vi "Main Editor UI.vi"() -> ()   [LabVIEW 2013, in "shared memory editor node.lvclass"]
doc: "This is the main view for configuration the behavior of a module in the DCAF standard editor."
uses:
  shared memory editor node.lvclass
  <vilib>/NI/Configuration Framework/Node/NodeRef.ctl
  <vilib>/NI/Configuration Framework/Node/NISE_CEF_Node.lvclass
  <vilib>/NI/AMC/Message Queue.ctl
  <vilib>/NI/AMC/Message.ctl
  <vilib>/NI/Tools/Keyed Array/KeyedArray.ctl
  <vilib>/NI/Configuration Framework/Node/UserEventRef.ctl
  <vilib>/NI/Configuration Framework/Controls/EventCluster.ctl
  <vilib>/NI/DCAF UI Toolkit/Controls/Configure.ctl
  <vilib>/NI/DCAF UI Toolkit/Controls/Add.ctl
  <vilib>/NI/DCAF UI Toolkit/Controls/Remove.ctl
  <vilib>/NI/Configuration Framework/Node/StopEvent.ctl
  <vilib>/NI/Configuration Framework/Node/RefreshUIEvent.ctl
  <vilib>/NI/Configuration Framework/Node/CacheState.ctl
  <vilib>/NI/Configuration Framework/Node/NodeChangeEvent.ctl
  <vilib>/NI/Tag Bus/tag/Data Type.ctl
  Permissions Enum.ctl
  <vilib>/NI/DCAF/Tag Editor Core/Table API/Available Tag Menu/channel action event.ctl
  <vilib>/NI/DCAF/Tag Editor Core/Table API/Available Tag Menu/dialog output action.ctl
  <vilib>/NI/Tag Bus Module Framework/channel/TBM channel.lvclass
  <vilib>/NI/Tag Bus/tag/tag descriptor.lvclass
  <vilib>/NI/DCAF/Tag Editor Core/Table API/Table Manager/Call Back Ref Type Def.ctl
  <vilib>/NI/DCAF/Tag Editor Core/Configuration Editor/Classes/Engine Parent/Engine Parent Editor Node.lvclass
  <vilib>/NI/DCAF/Tag Editor Core/Configuration Editor/Classes/Module editor node/module editor node.lvclass
  <vilib>/NI/DCAF/Tag Editor Core/Table API/Table Manager/references.ctl
  <vilib>/NI/DCAF/Tag Editor Core/Table API/Listbox/Multi Column Listbox.lvclass
  <vilib>/Utility/miscctls.llb/LVPositionTypeDef.ctl
  <vilib>/NI/DCAF/Tag Editor Core/Configuration Editor/Classes/Engine Parent/read engine configuration.vi
  <vilib>/NI/Configuration Framework/NISE_CEF_TreeControl.lvlib
  <vilib>/NI/Tools/Keyed Array/Tools_KeyedArray.lvlib
  <vilib>/NI/AMC/AMC.lvlib
  <vilib>/NI/DCAF/Tag Editor Core/Table API/Table Manager.lvlib
  <vilib>/NI/DCAF/Tag Editor Core/Table API/Table Manager/Table Manager.lvclass
  <vilib>/NI/DCAF UI Toolkit/Controls/DCAF UI Elements.lvlib
panel:
  in  "user event out":refnum<user-event>
  in  "Permissions":T1
  in  "data type":T2
  in  "node change":T3
  in  "cache state":T4
  in  "refresh UI":T5
  in  "stop event":T6
  in  "Tab Control":T7(tab)
  in  "Remove Button":T8
  in  "Add Button":T9
  in  "Table":i32(listbox)
  in  "settings":T10
  in  "output file string":string caption="output file string (data engine input)"
  in  "input file string":string caption="input file string (data engine output)"
  in  "name string":string caption="name string (optional)"
  in  "C header file directory":path
  in  "C header":bool
  in  "user event":T11
  in  "main queue":T12
  in  "node ref":T13
  # "Directories relative to engine root (/dev/shm/<EngineName>)"
  # "It is recommended that directory names be chosen to reflect the perspective of an the external process or application that accesses the file in shared memory.\n\nExample: A C application running in parallel to the DCAF based LabVIEW Real-Time EXE will view any folder that it writes to (which are read by the data engine) to be an \"output\" folder."
  # "C Header File Generation"
  # "Generate a C header file in a \"C header file directory\" which contains shared memory mapping information for use in C applications. The default C header file name will use the configuration file name and add optional user \"name string\" text: \n\nConfigurationFileName<_NameString>.h\n\nNote: The user will override the file name format if the \".h\" file extension is included."
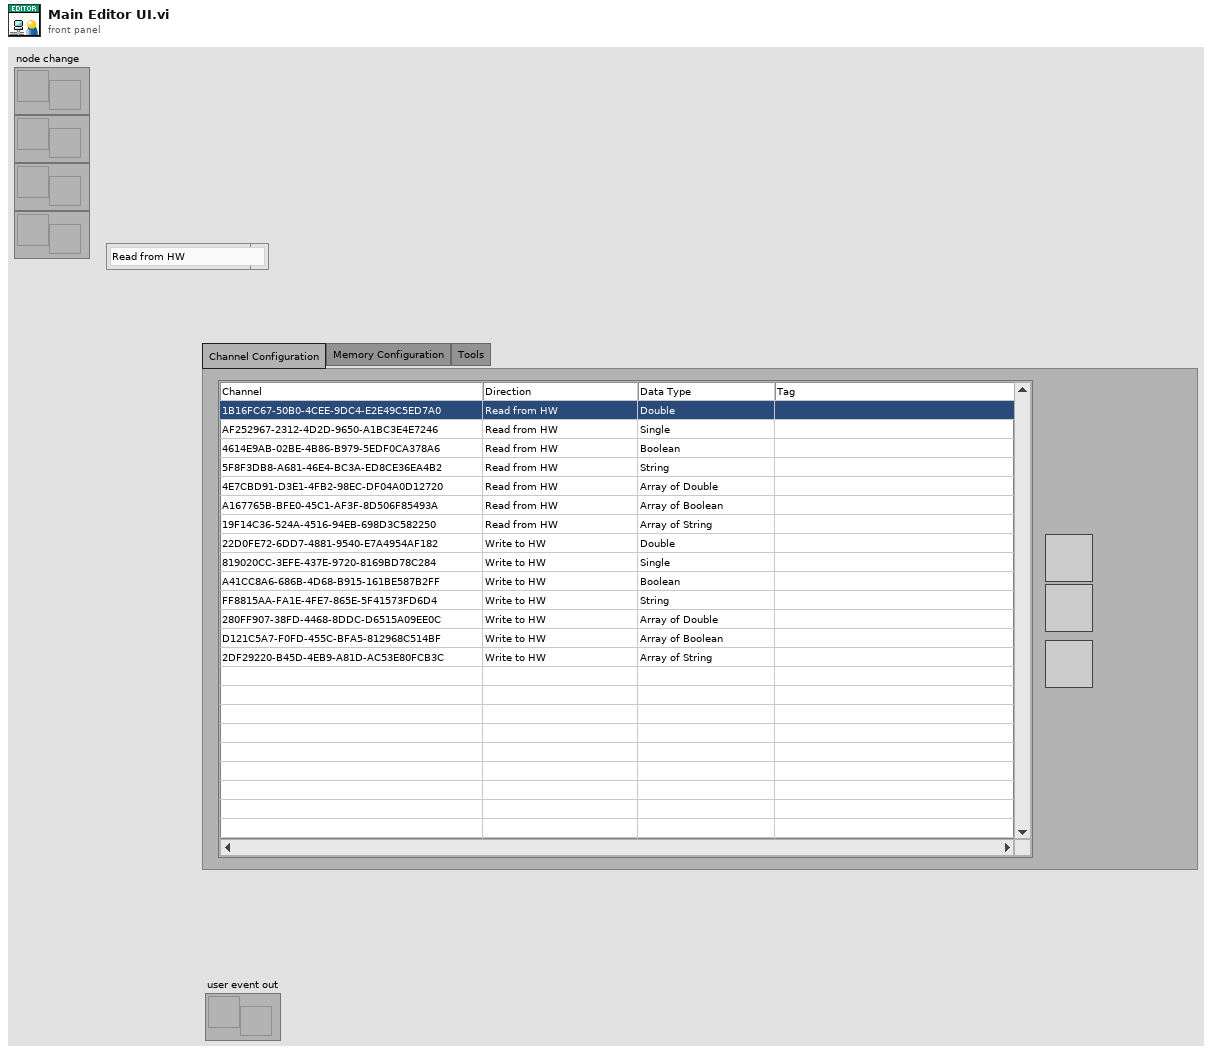
[diagram p1: front panel]
types:
  T1 = typedef "shared memory editor node.lvclass/Permissions Enum.ctl" = enum16{"Read from HW", "Write to HW"}
  T2 = typedef "tag bus.lvlib/tag descriptor.lvclass/Data Type.ctl" = enum16{"Double", "Single", "I64", "I32", "I16", "I8", "U64", "U32", "U16", "U8", "Boolean", "String", "Array of Double", "Array of Single", "Array of I64", "Array of I32", "Array of I16", "Array of I8", "Array of U64", "Array of U32", "Array of U16", "Array of U8", "Array of Boolean", "Array of String"}
  T3 = typedef "NISE_CEF_Node.lvclass/NodeChangeEvent.ctl" = refnum<user-event>
  T4 = typedef "NISE_CEF_Node.lvclass/CacheState.ctl" = refnum<user-event>
  T5 = typedef "NISE_CEF_Node.lvclass/RefreshUIEvent.ctl" = refnum<user-event>
  T6 = typedef "NISE_CEF_Node.lvclass/StopEvent.ctl" = refnum<user-event>
  T7 = enum32{"Channel Configuration", "Memory Configuration", "Tools"}
  T8 = typedef "DCAF UI Elements.lvlib/Remove.ctl" = bool
  T9 = typedef "DCAF UI Elements.lvlib/Add.ctl" = bool
  T10 = typedef "DCAF UI Elements.lvlib/Configure.ctl" = bool
  T11 = typedef "NISE_CEF_Node.lvclass/UserEventRef.ctl" = refnum<user-event>
  T12 = typedef "AMC.lvlib/Message Queue.ctl" = refnum<queue>
  T13 = typedef "NISE_CEF_Node.lvclass/NodeRef.ctl" = refnum<data-value>
  T14 = typedef "Table Manager.lvlib/Table Manager.lvclass/references.ctl" = cluster{"stop event":T6, "refresh UI":T5, "cache state":T4, "node change":T3, "user event out":refnum<user-event>, "main queue":T12, "user event":T11}
  T15 = typedef "LVPositionTypeDef.ctl" = cluster{"Left":i32, "Top":i32}
  T16 = typedef "Table Manager.lvlib/Table Manager.lvclass/object ref.ctl" = cluster{"engine":refnum<data-value>, "Node Ref":refnum<data-value>}
  T17 = typedef "Table Manager.lvlib/Column.lvclass/Column Descriptor.ctl" = cluster{"name":string, "caption":string, "Column Type":T18, "Params":string, "AutoSizeMode":i32, "FillWeight":sgl, "MinWidth":u32, "tooltip":string, "Enum Reference":refnum<vi>, "Channel suffix":string, "Read Only":bool, "Call Back VI":T19, "DT Dependency":i32, "name dependency":i32, "data type":T2, "Custom Column":refnum<class "Column.lvclass">}
  T18 = typedef "Table Manager.lvlib/Column.lvclass/Column Type.ctl" = enum16{"String", "Mapping", "Enum", "Custom"}
  T19 = typedef "Table Manager.lvlib/Table Manager.lvclass/Call Back Ref Type Def.ctl" = refnum<vi>
  T20 = typedef "Table Manager.lvlib/Table Manager.lvclass/Table Events.ctl" = cluster{"Menu Selection":refnum<user-event>}
  T21 = enum8{"Enabled", "Disabled", "Disabled and Grayed Out"}
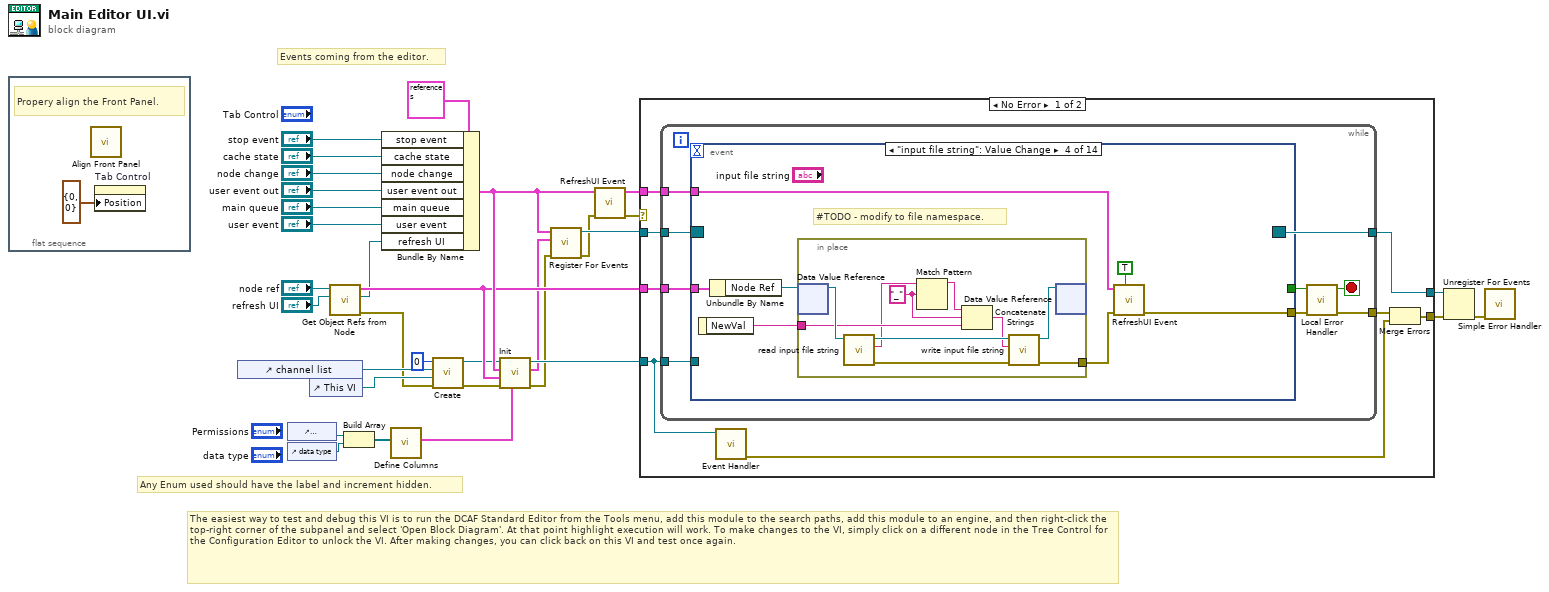
[diagram p0: block diagram]
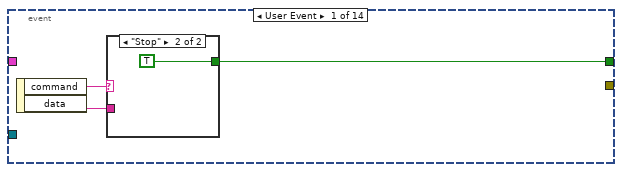
[diagram p2: hidden frame]
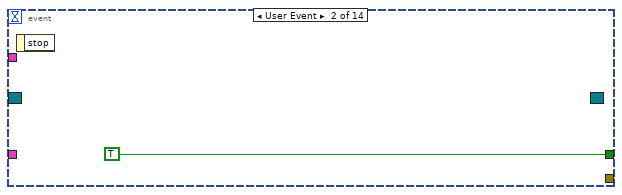
[diagram p4: hidden frame]
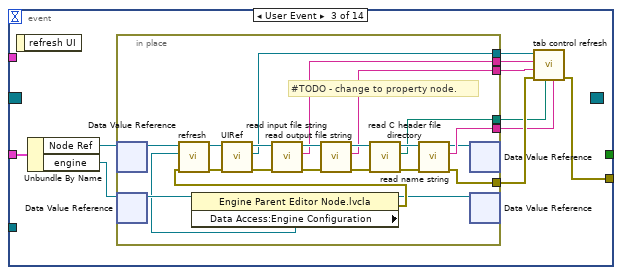
[diagram p5: hidden frame]
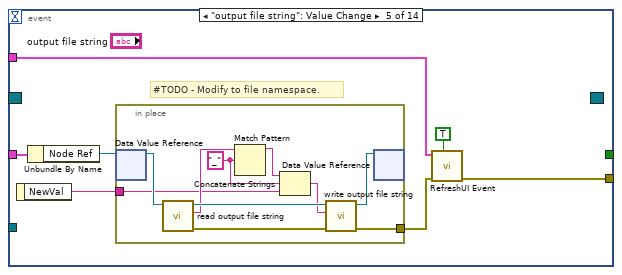
[diagram p6: hidden frame]
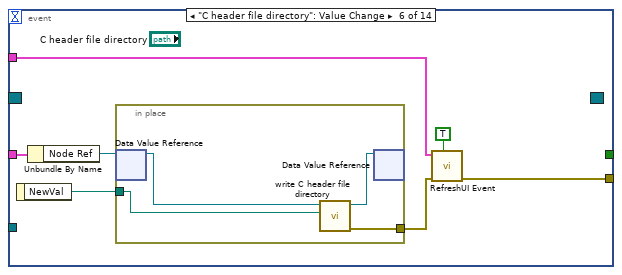
[diagram p7: hidden frame]
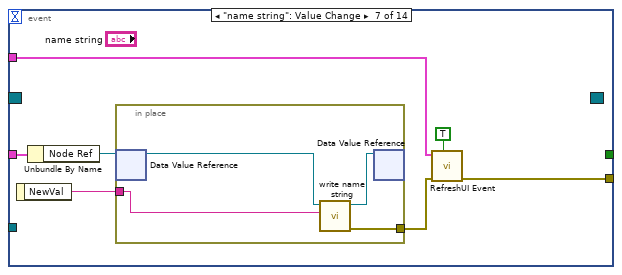
[diagram p8: hidden frame]
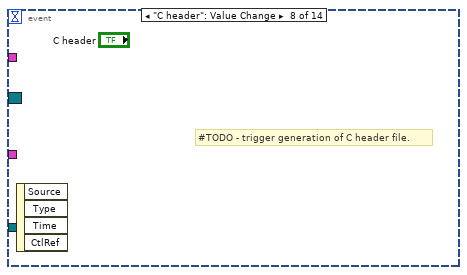
[diagram p9: hidden frame]
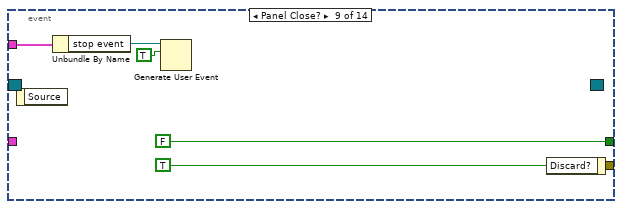
[diagram p10: hidden frame]
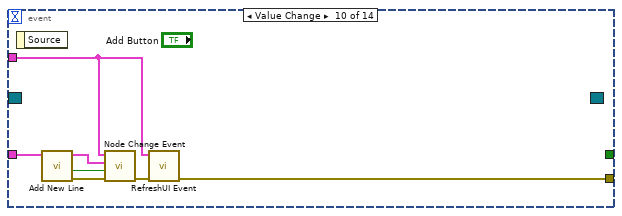
[diagram p11: hidden frame]
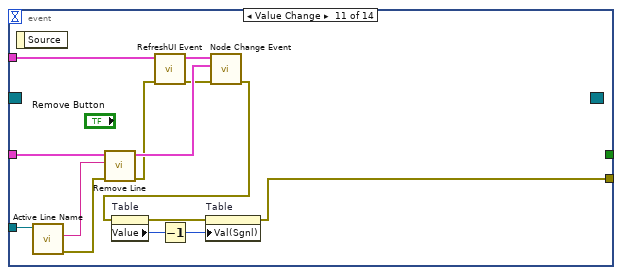
[diagram p12: hidden frame]
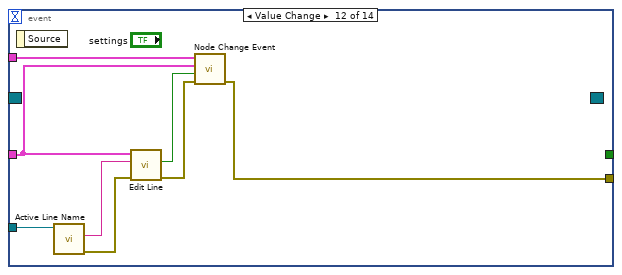
[diagram p13: hidden frame]
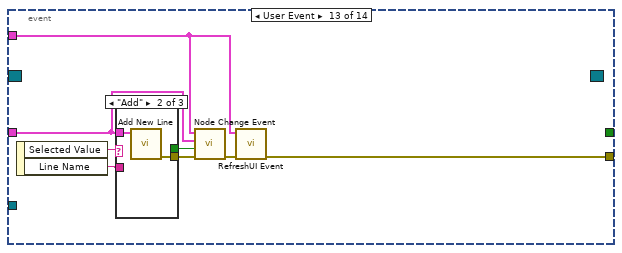
[diagram p14: hidden frame]
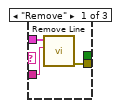
[diagram p15: hidden frame]
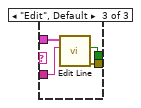
[diagram p16: hidden frame]
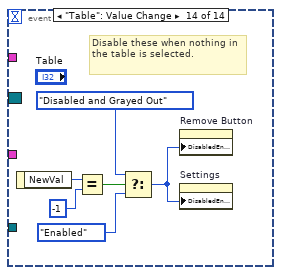
[diagram p17: hidden frame]
diagram:
  # "The easiest way to test and debug this VI is to run the DCAF Standard Editor from the Tools menu, add this module to the search paths, add this module to an engine, and then right-click the top-right corner of the subpanel and select 'Open Block Diagram'. At that point highlight execution will work. To make changes to the VI, simply click on a different node in the Tree Control for the Configuration Editor to unlock the VI. After making changes, you can click back on this VI and test once again."
  # "Any Enum used should have the label and increment hidden."
  # "Events coming from the editor."
  n1 = flat-sequence {
    frame #0 {
      # "Propery align the Front Panel."
      n2 = call <vilib>:"Align Front Panel.vi"() -> ()  [unwired: 10 in, 2 out]
      n3 = property on="Tab Control" class="TabCtl (strict)"("Position"=T15 {"Left"=0, "Top"=0}) -> ()  [unwired: 2 in, 2 out]
    }
  }
  n4 = control-ref of="channel list"() -> (w8:refnum<vi>)
  n5 = control-ref of="Permissions"() -> (w18:refnum<vi>)
  n6 = control-ref of="data type"() -> (w17:refnum<vi>)
  n7 = control-ref of="This VI"() -> (w6:refnum<vi>)
  n8 = call "Get Object Refs from Node.vi"("Refresh UI"="refresh UI", "Data Value Reference in"="node ref") -> ("error out"=w3:errorcluster, "Refresh UI out"=w1:T5, "References"=w15:T16)  [unwired: 7 in]
  n9 = Build Array(w18, w17) -> (w16:refnum<vi>[])
  n10 = Bundle By Name(cluster=T14 {"stop event"=refnum, "refresh UI"=refnum, "cache state"=refnum, "node change"=refnum, "user event out"=refnum, "main queue"=refnum, "user event"=refnum} ("References"), "stop event"="stop event", "cache state"="cache state", "node change"="node change", "user event out"="user event out", "main queue"="main queue", "user event"="user event", "refresh UI"=w1) -> (w19:T14)
  n11 = call "Define Columns.vi"("Enum Array"=w16) -> ("Column Definition"=w21:T17[])  [unwired: 10 in]
  n12 = call <vilib>:"Create.vi"("error in (no error)"=w3, "Top VI"=w6, "Listbox"=w8, "Index"=0) -> ("error out"=w4:errorcluster, "reference out"=w5:refnum<class "Multi Column Listbox.lvclass">)  [unwired: 6 in]
  n13 = call-dynamic "Init.vi"("Column Descriptors"=w21, "error in (no error)"=w4, "Node object refs"=w15, "Event References"=w19, "Multi Column Listbox in"=w5) -> ("error out"=w10:errorcluster, "Table Events"=w9:T20, "Multi Column Listbox out"=w14:refnum<class "Multi Column Listbox.lvclass">)  [unwired: 4 in]
  n14 = call "Register For Events.vi"("error in"=w10, "Table Events"=w9, "References"=w19) -> ("error out"=w12:errorcluster, "Event Registration Refnum"=w22:refnum<event-registration>)  [unwired: 7 in]
  n15 = call "RefreshUI Event.vi"("error in (no error)"=w12, "References in"=w19) -> ("error out"=w11:errorcluster, "References out"=w20:T14)  [unwired: 8 in]
  n16 = case shown="No Error" w11 {
    selector: w11 -> [_ w200]
    tunnel: w22 -> [w41 w199]
    tunnel: [w40 w199] -> w32
    tunnel: [w34 w200] -> w31
    tunnel: w20 -> [w39 _]
    tunnel: w15 -> [w38 _]
    tunnel: w14 -> [w37 _]
    frame No Error {
      n17 = while {
        tunnel: w41 -> [w50]
        tunnel: [w49] -> w40
        tunnel: [w46] -> w35
        tunnel: w39 -> [w44]
        tunnel: w38 -> [w43]
        tunnel: w37 -> [w42]
        stop <- w48 stop-if-true
        n18 = event shown="[3] \"input file string\": Value Change" {
          selector: w50 -> [_ _ _ _ _ _ _ _ _ _ _ _ _ _]
          dyn-events: [_ _ _ _ _ _ _ _ _ _ _ _ _ _] -> w49
          timeout: _ -> [_ _ _ _ _ _ _ _ _ _ _ _ _ _]
          tunnel: [w53 TRUE _ _ _ _ _ _ FALSE _ _ _ _ _] -> w47
          tunnel: [_ _ w61 w91 w108 w125 w136 _ _ w149 w156 w173 w181 _] -> w45
          tunnel: w44 -> [_ _ _ w90 w107 w124 w135 _ w145 w153 w167 w175 w177 _]
          tunnel: w43 -> [_ _ w65 w94 w111 w128 w139 _ _ w154 w166 w171 w178 _]
          tunnel: w42 -> [_ _ _ _ _ _ _ _ _ _ w162 w172 _ _]
          event User Event {
            n19 = event-data() -> ("command"=w52:string, "data"=w51:string)  [unwired: 1 in]
            n20 = case shown="\"Stop\"" w52 {
              tunnel: [_ TRUE] -> w53
              tunnel: w51 -> [_ _]
              frame Default {
              }
              frame "Stop" {
              }
            }
          }
          event User Event {
            n21 = event-data() -> ()  [unwired: 1 in, 1 out]
          }
          event User Event {
            n22 = event-data() -> ()  [unwired: 1 in, 1 out]
            n23 = Unbundle By Name(w65) -> ("Node Ref"=w64:refnum<data-value>, "engine"=w63:refnum<data-value>)
            n24 = in-place {
              in-place-border: [w84] -> w62
              in-place-border: [w77] -> w56
              in-place-border: [w71] -> w60
              in-place-border: [w70] -> w59
              in-place-border: [w69] -> w58
              in-place-border: [w68] -> w57
              # "#TODO - change to property node."
              n25 = in-place-dvr #1(w64) -> (w82:refnum<class "module editor node.lvclass">)  [unwired: 1 out]
              n26 = in-place-dvr #2(w63) -> (w87:refnum<class "Engine Parent Editor Node.lvclass">)  [unwired: 1 out]
              n27 = property class="Engine Parent Editor Node.lvcla"(reference=w87) -> (reference out=w66:refnum<class "Engine Parent Editor Node.lvclass">, error out=w79:errorcluster, "Data Access:Engine Configuration"=w80:refnum<class "engine configuration.lvclass">)  [unwired: 1 in]
              n28 = call-dynamic "refresh.vi"("error in (no error)"=w79, "Engine Configuration In"=w80, "Module Editor Node In"=w82) -> ("error out"=w76:errorcluster, "Module Editor Node Out"=w81:refnum<class "module editor node.lvclass">)  [unwired: 6 in, 1 out]
              n29 = call-dynamic "UIRef.vi"("error in"=w76, "node in"=w81) -> ("error out"=w75:errorcluster, "VI refnum"=w77:refnum<vi>, "node out"=w78:refnum<class "module editor node.lvclass">)  [unwired: 7 in]
              n30 = call "read input file string.vi"("error in"=w75, "shared memory editor node"=w78) -> ("error out"=w86:errorcluster, "input file string"=w71:string, "shared memory editor node out"=w74:refnum<class "module editor node.lvclass">)  [unwired: 7 in]
              n31 = call "read output file string.vi"("error in"=w86, "shared memory editor node"=w74) -> ("error out"=w85:errorcluster, "output file string"=w70:string, "shared memory editor node out"=w73:refnum<class "module editor node.lvclass">)  [unwired: 7 in]
              n32 = call "read C header file directory.vi"("error in"=w85, "shared memory editor node"=w73) -> ("error out"=w83:errorcluster, "C header file directory"=w69:path, "shared memory editor node out"=w72:refnum<class "module editor node.lvclass">)  [unwired: 7 in]
              n33 = call "read name string.vi"("error in"=w83, "shared memory editor node"=w72) -> ("error out"=w84:errorcluster, "name string"=w68:string, "shared memory editor node out"=w67:refnum<class "module editor node.lvclass">)  [unwired: 7 in]
              n34 = in-place-dvr #1(w67) -> ()  [unwired: 2 out]
              n35 = in-place-dvr #2(w66) -> ()  [unwired: 2 out]
            }
            n36 = call "tab control refresh.vi"("name string"=w57, "C header file directory"=w58, "error in"=w62, "output file string"=w59, "input file string"=w60, "VI reference"=w56) -> ("error out"=w61:errorcluster)  [unwired: 5 in]
          }
          event "input file string": Value Change {
            # "#TODO - modify to file namespace."
            n37 = event-data() -> ("NewVal"=w92:string)  [unwired: 1 in]
            n38 = Unbundle By Name(w94) -> ("Node Ref"=w93:refnum<data-value>)
            n39 = in-place {
              in-place-border: w92 -> [w97]
              in-place-border: [w100] -> w88
              w98 = "_" ("string")
              n40 = in-place-dvr #3(w93) -> (w103:refnum<class "module editor node.lvclass">)  [unwired: 1 out]
              n41 = call "read input file string.vi"("shared memory editor node"=w103) -> ("error out"=w101:errorcluster, "input file string"=w95:string, "shared memory editor node out"=w102:refnum<class "module editor node.lvclass">)  [unwired: 8 in]
              n42 = Match Pattern(string=w95, regular expression=w98) -> (before substring=w99:string)  [unwired: 1 in, 3 out]
              n43 = Concatenate Strings(w99, w98, w97) -> (w96:string)
              n44 = call "write input file string.vi"("error in"=w101, "input file string"=w96, "shared memory editor node"=w102) -> ("error out"=w100:errorcluster, "shared memory editor node out"=w104:refnum<class "module editor node.lvclass">)  [unwired: 7 in]
              n45 = in-place-dvr #3(w104) -> ()  [unwired: 2 out]
            }
            n46 = call "RefreshUI Event.vi"("Refresh (T)"=TRUE, "error in (no error)"=w88, "References in"=w90) -> ("error out"=w91:errorcluster)  [unwired: 7 in, 1 out]
          }
          event "output file string": Value Change {
            # "#TODO - Modify to file namespace."
            n47 = event-data() -> ("NewVal"=w109:string)  [unwired: 1 in]
            n48 = Unbundle By Name(w111) -> ("Node Ref"=w110:refnum<data-value>)
            n49 = in-place {
              in-place-border: w109 -> [w115]
              in-place-border: [w117] -> w105
              w113 = "_" ("string")
              n50 = in-place-dvr #4(w110) -> (w120:refnum<class "module editor node.lvclass">)  [unwired: 1 out]
              n51 = call "read output file string.vi"("shared memory editor node"=w120) -> ("error out"=w118:errorcluster, "output file string"=w116:string, "shared memory editor node out"=w119:refnum<class "module editor node.lvclass">)  [unwired: 8 in]
              n52 = Match Pattern(string=w116, regular expression=w113) -> (before substring=w114:string)  [unwired: 1 in, 3 out]
              n53 = Concatenate Strings(w114, w113, w115) -> (w112:string)
              n54 = call "write output file string.vi"("error in"=w118, "output file string"=w112, "shared memory editor node"=w119) -> ("error out"=w117:errorcluster, "shared memory editor node out"=w121:refnum<class "module editor node.lvclass">)  [unwired: 7 in]
              n55 = in-place-dvr #4(w121) -> ()  [unwired: 2 out]
            }
            n56 = call "RefreshUI Event.vi"("Refresh (T)"=TRUE, "error in (no error)"=w105, "References in"=w107) -> ("error out"=w108:errorcluster)  [unwired: 7 in, 1 out]
          }
          event "C header file directory": Value Change {
            n57 = event-data() -> ("NewVal"=w126:path)  [unwired: 1 in]
            n58 = Unbundle By Name(w128) -> ("Node Ref"=w127:refnum<data-value>)
            n59 = in-place {
              in-place-border: w126 -> [w129]
              in-place-border: [w131] -> w122
              n60 = in-place-dvr #5(w127) -> (w130:refnum<class "module editor node.lvclass">)  [unwired: 1 out]
              n61 = call "write C header file directory.vi"("C header file directory"=w129, "shared memory editor node"=w130) -> ("error out"=w131:errorcluster, "shared memory editor node out"=w132:refnum<class "module editor node.lvclass">)  [unwired: 8 in]
              n62 = in-place-dvr #5(w132) -> ()  [unwired: 2 out]
            }
            n63 = call "RefreshUI Event.vi"("Refresh (T)"=TRUE, "error in (no error)"=w122, "References in"=w124) -> ("error out"=w125:errorcluster)  [unwired: 7 in, 1 out]
          }
          event "name string": Value Change {
            n64 = event-data() -> ("NewVal"=w137:string)  [unwired: 1 in]
            n65 = Unbundle By Name(w139) -> ("Node Ref"=w138:refnum<data-value>)
            n66 = in-place {
              in-place-border: w137 -> [w141]
              in-place-border: [w142] -> w133
              n67 = in-place-dvr #6(w138) -> (w140:refnum<class "module editor node.lvclass">)  [unwired: 1 out]
              n68 = call "write name string.vi"("name string"=w141, "shared memory editor node"=w140) -> ("error out"=w142:errorcluster, "shared memory editor node out"=w143:refnum<class "module editor node.lvclass">)  [unwired: 8 in]
              n69 = in-place-dvr #6(w143) -> ()  [unwired: 2 out]
            }
            n70 = call "RefreshUI Event.vi"("Refresh (T)"=TRUE, "error in (no error)"=w133, "References in"=w135) -> ("error out"=w136:errorcluster)  [unwired: 7 in, 1 out]
          }
          event "C header": Value Change {
            # "#TODO - trigger generation of C header file."
            n71 = event-data() -> ()  [unwired: 1 in, 4 out]
          }
          event Panel Close? {
            n72 = event-data() -> ()  [unwired: 1 in, 1 out]
            n73 = Unbundle By Name(w145) -> ("stop event"=w144:T6)
            n74 = Generate User Event(user event=w144, event data cluster=TRUE ("event data")) -> ()  [unwired: 2 in, 2 out]
            n75 = event-data("Discard?"=TRUE) -> ()  [unwired: 1 in, 1 out]
          }
          event Value Change {
            n76 = event-data() -> ()  [unwired: 1 in, 1 out]
            n77 = call "Add New Line.vi"("objects"=w154) -> ("error out"=w152:errorcluster, "success"=w150:bool)  [unwired: 8 in, 1 out]
            n78 = call "Node Change Event.vi"("error in (no error)"=w152, "Send (T)"=w150, "objects"=w154, "References in"=w153) -> ("error out"=w151:errorcluster)  [unwired: 7 in]
            n79 = call "RefreshUI Event.vi"("error in (no error)"=w151, "References in"=w153) -> ("error out"=w149:errorcluster)  [unwired: 8 in, 1 out]
          }
          event Value Change {
            n80 = event-data() -> ()  [unwired: 1 in, 1 out]
            n81 = call-dynamic "Active Line Name.vi"("Multi Column Listbox in"=w162) -> ("error out"=w160:errorcluster, "Active Line Name"=w161:string)  [unwired: 8 in, 1 out]
            n82 = call "Remove Line.vi"("error in"=w160, "Active Line Name"=w161, "Objects"=w166) -> ("error out"=w163:errorcluster)  [unwired: 8 in]
            n83 = call "RefreshUI Event.vi"("error in (no error)"=w163, "References in"=w167) -> ("error out"=w165:errorcluster, "References out"=w164:T14)  [unwired: 8 in]
            n84 = call "Node Change Event.vi"("error in (no error)"=w165, "objects"=w166, "References in"=w164) -> ("error out"=w157:errorcluster)  [unwired: 8 in]
            n85 = property on="Table" class="MCListbox (strict)"(error in=w157) -> (error out=w155:errorcluster, "Value"=w158:i32)  [unwired: 1 in, 1 out]
            n86 = Decrement(x=w158) -> (x-1=w159:i32)
            n87 = property on="Table" class="MCListbox (strict)"(error in=w155, "Val(Sgnl)"=w159) -> (error out=w156:errorcluster)  [unwired: 1 in, 1 out]
          }
          event Value Change {
            n88 = event-data() -> ()  [unwired: 1 in, 1 out]
            n89 = call-dynamic "Active Line Name.vi"("Multi Column Listbox in"=w172) -> ("error out"=w169:errorcluster, "Active Line Name"=w170:string)  [unwired: 8 in, 1 out]
            n90 = call "Edit Line.vi"("error in"=w169, "Line Name"=w170, "References"=w171) -> ("error out"=w174:errorcluster, "change?"=w168:bool)  [unwired: 7 in]
            n91 = call "Node Change Event.vi"("error in (no error)"=w174, "Send (T)"=w168, "objects"=w171, "References in"=w175) -> ("error out"=w173:errorcluster)  [unwired: 7 in]
          }
          event User Event {
            n92 = event-data() -> ("Selected Value"=w183:string, "Line Name"=w180:string)  [unwired: 1 in]
            n93 = case shown="\"Add\"" w183 {
              tunnel: w180 -> [w186 _ w192]
              tunnel: w178 -> [w185 w188 w191]
              tunnel: [w184 w187 w190] -> w179
              tunnel: [_ _ w189] -> w176
              frame "Remove" {
                n94 = call "Remove Line.vi"("Active Line Name"=w186, "Objects"=w185) -> ("error out"=w184:errorcluster)  [unwired: 9 in]
              }
              frame "Add" {
                n95 = call "Add New Line.vi"("objects"=w188) -> ("error out"=w187:errorcluster)  [unwired: 8 in, 2 out]
              }
              frame "Edit", Default {
                n96 = call "Edit Line.vi"("Line Name"=w192, "References"=w191) -> ("error out"=w190:errorcluster, "change?"=w189:bool)  [unwired: 8 in]
              }
            }
            n97 = call "Node Change Event.vi"("error in (no error)"=w179, "Send (T)"=w176, "objects"=w178, "References in"=w177) -> ("error out"=w182:errorcluster)  [unwired: 7 in]
            n98 = call "RefreshUI Event.vi"("error in (no error)"=w182, "References in"=w177) -> ("error out"=w181:errorcluster)  [unwired: 8 in, 1 out]
          }
          event "Table": Value Change {
            # "Disable these when nothing in the table is selected."
            n99 = event-data() -> ("NewVal"=w198:i32)  [unwired: 1 in]
            n100 = Equal?(x=w198, y=-1) -> (x = y?=w196:bool)
            n101 = Select(t=T21."Disabled and Grayed Out" ("Disabled"), s=w196, f=T21."Enabled") -> (s? t:f=w194:T21)
            n102 = property on="Remove Button" class="Bool"("DisabledEnum"=w194) -> ()  [unwired: 2 in, 2 out]
            n103 = property on="Settings" class="Bool"("DisabledEnum"=w194) -> ()  [unwired: 2 in, 2 out]
          }
        }
        n104 = call "Local Error Handler.vi"("error in"=w45, "Stop in"=w47) -> ("error out"=w46:errorcluster, "Stop out"=w48:bool)  [unwired: 8 in]
      }
      n105 = call-dynamic "Event Handler.vi"("Listbox in"=w37) -> ("error out"=w36:errorcluster)  [unwired: 9 in, 1 out]
      n106 = Merge Errors(w35, w36) -> (w34:errorcluster)
    }
    frame Error {
    }
  }
  n107 = Unregister For Events(event registration refnum=w32, error in=w31) -> (error out=w30:errorcluster)
  n108 = call <vilib>:"Simple Error Handler.vi"("error in (no error)"=w30) -> ()  [unwired: 4 in, 5 out]
